vi "SaveInit.vi"(11 "Name":string) -> (3 "TDMSFile":refnum<k34>)   [LabVIEW 2019]
panel:
  # "This Vi opens the TDMS files in which the setting and data is saved."
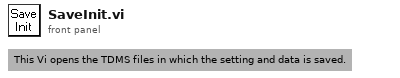
[diagram p1: front panel]
types:
  T1 = enum16{"open", "open or create", "create or replace", "create", "open (read-only)"}
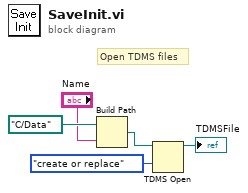
[diagram p0: block diagram]
diagram:
  # "Open TDMS files"
  n1 = Build Path(base path=path "C:/Data" ("file path"), name or relative path="Name") -> (appended path=w3:path)
  n2 = TDMS Open(10:T1."create or replace" ("operation (0:open)"), 11:w3) -> (3:→"TDMSFile":refnum<k34>)  [unwired: 5 in, 1 out]
